vi "Create.vi"(8 "error in (no error)":errorcluster, 10 "This Actor":T1) -> (0 "error out":errorcluster, 3 "Protected Actor Handle out":refnum<class "Protected Actor Handle.lvclass">)   [LabVIEW 2020, in "Actor Framework.lvlib" / "Protected Actor Handle.lvclass"]
doc: "Given the information about an actor, provided by the debug layer of the Actor Framework, this VI creates an actor handle that an attached debugger can use for limited manipulation of the running actor."
uses:
  Protected Actor Handle.lvclass
  Support/This Actor.ctl
  Message Enqueuer/Message Enqueuer.lvclass
  Protected Actor Handle.lvclass/Protected Actor Handle.ctl
  Actor Framework.lvlib
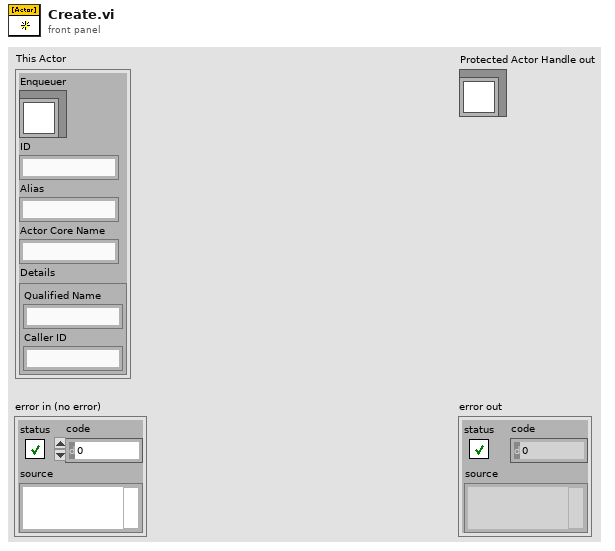
[diagram p1: front panel]
types:
  T1 = typedef "Actor Framework.lvlib/This Actor.ctl" = cluster{"Enqueuer":refnum<class "Message Enqueuer.lvclass">, "ID":string, "Alias":string, "Actor Core Name":string, "Details":cluster{"Qualified Name":string, "Caller ID":string}}
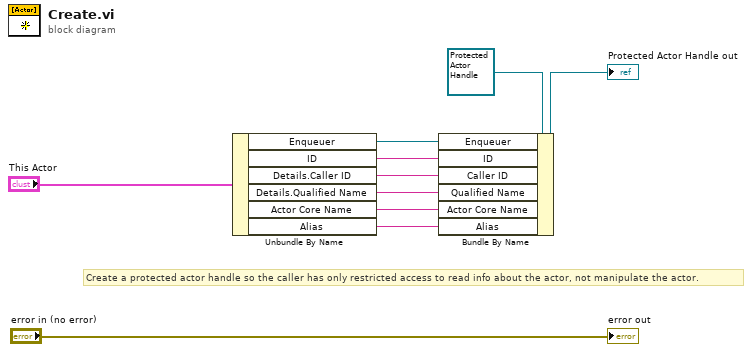
[diagram p0: block diagram]
diagram:
  # "Create a protected actor handle so the caller has only restricted access to read info about the actor, not manipulate the actor."
  n1 = Unbundle By Name("This Actor") -> ("Enqueuer"=w6:refnum<class "Message Enqueuer.lvclass">, "ID"=w5:string, "Details.Caller ID"=w4:string, "Details.Qualified Name"=w3:string, "Actor Core Name"=w2:string, "Alias"=w1:string)
  n2 = Bundle By Name(cluster=refnum<class "Protected Actor Handle.lvclass"> refnum ("Protected Actor Handle in"), "Enqueuer"=w6, "ID"=w5, "Caller ID"=w4, "Qualified Name"=w3, "Actor Core Name"=w2, "Alias"=w1) -> (→"Protected Actor Handle out":refnum<class "Protected Actor Handle.lvclass">)
  "error out" <- "error in (no error)"
